vi "Move.vi"(8 "error in (no error)":errorcluster, 9 "Absolute (T)":bool=TRUE, 10 "Point":refnum<class "Point.lvclass">, 11 "Circle in":refnum<class "Circle.lvclass">) -> (0 "error out":errorcluster, 3 "Circle out":refnum<class "Circle.lvclass">)   [LabVIEW 2021, in "Picture2D.lvlib" / "Circle.lvclass"]
uses:
  Circle.lvclass
  Shape/Shape.lvclass
  Point/Point.lvclass
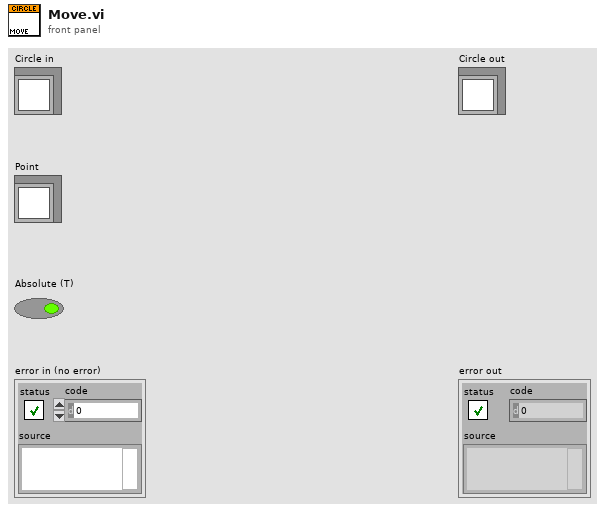
[diagram p1: front panel]
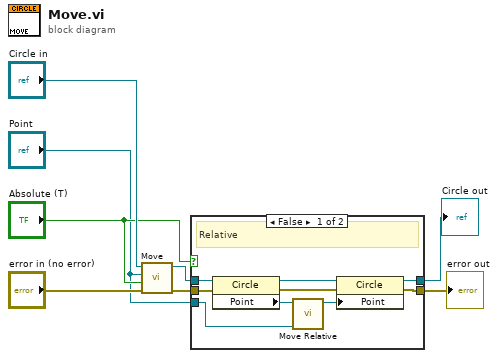
[diagram p0: block diagram]
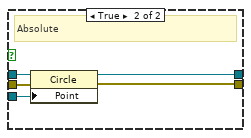
[diagram p2: hidden frame]
diagram:
  n1 = call-parent "Move.vi"("error in (no error)"="error in (no error)", "Absolute (T)"="Absolute (T)", "Point"="Point", "Shape in"="Circle in") -> ("error out"=w2:errorcluster, "Shape out"=w6:refnum<class "Circle.lvclass">)  [unwired: 6 in]
  n2 = case shown="False" "Absolute (T)" {
    tunnel: w6 -> [w16 w22]
    tunnel: [w12 w21] -> w5
    tunnel: "Point" -> [w17 w20]
    tunnel: w2 -> [w11 w19]
    tunnel: [w9 w18] -> w1
    frame False {
      # "Relative"
      n3 = property class="Circle"(reference=w16, error in=w11) -> (reference out=w13:refnum<class "Circle.lvclass">, error out=w10:errorcluster, "Point"=w15:refnum<class "Point.lvclass">)
      n4 = call "Move Relative.vi"("Move"=w17, "Point"=w15) -> ("New Point"=w14:refnum<class "Point.lvclass">)  [unwired: 9 in]
      n5 = property class="Circle"(reference=w13, error in=w10, "Point"=w14) -> (reference out=w12:refnum<class "Circle.lvclass">, error out=w9:errorcluster)
    }
    frame True {
      # "Absolute"
      n6 = property class="Circle"(reference=w22, error in=w19, "Point"=w20) -> (reference out=w21:refnum<class "Circle.lvclass">, error out=w18:errorcluster)
    }
  }
  "error out" <- w1
  "Circle out" <- w5
